vi "SET FRONT FACE.vi"(10 "front face":T1) -> ()   [LabVIEW 2023]
uses:
  ctrl defs/ctrl FRONT FACE selector.ctl
  Global odometry.vi
  <vilib>/Rock Robotics/Network Tables/NT Write String.vi
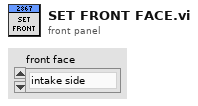
[diagram p1: front panel]
types:
  T1 = typedef "ctrl FRONT FACE selector.ctl" = enum16{"intake side", "shooter side"}
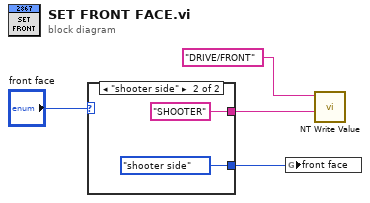
[diagram p0: block diagram]
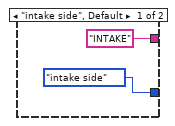
[diagram p2: hidden frame]
diagram:
  n1 = case shown="\"shooter side\"" "front face" {
    tunnel: ["INTAKE" ("value") "SHOOTER" ("value")] -> w2
    tunnel: [ctrl_FRONT_FACE_selector."intake side" ("front face") ctrl_FRONT_FACE_selector."shooter side" ("front face")] -> w1
    frame "intake side", Default {
    }
    frame "shooter side" {
    }
  }
  n2 = global write "Global odometry.vi" "front face"(w1) -> ()
  n3 = call-poly <vilib>:"NT Write Value.vi"("value"=w2, "name"="DRIVE/FRONT") -> ()  [unwired: 9 in, 1 out]
